vi "Img Write Ref Value.vi"(8 "error in (no error)":errorcluster, 10 "Image":variant, 11 "Image Ref":refnum<vi>) -> (0 "error out":errorcluster)   [LabVIEW 2018, in "Image Process.lvclass"]
uses:
  Image Process.lvclass
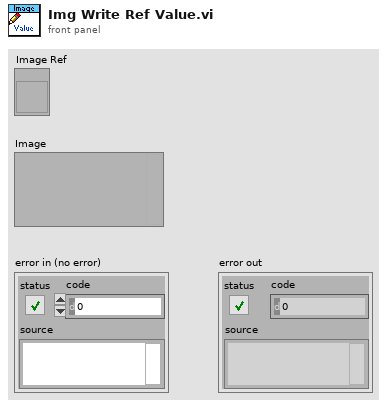
[diagram p1: front panel]
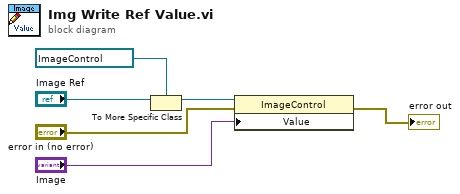
[diagram p0: block diagram]
diagram:
  n1 = To More Specific Class(target class=refnum<vi> refnum ("reference"), reference="Image Ref") -> (specific class reference=w4:refnum<vi>)  [unwired: 1 in, 1 out]
  n2 = property class="ImageControl"(reference=w4, error in="error in (no error)", "Value"="Image") -> (error out=→"error out":errorcluster)  [unwired: 1 out]
